vi "Constructor.vi"(8 "error in (no error)":errorcluster, 10 "Configuration.Application":enum16{"TC", "FP"}(ring), 11 "FP-TC-Shared in":refnum<class "FP-TC-Shared.lvclass">) -> (0 "error out":errorcluster, 3 "FP-TC-Shared out":refnum<class "FP-TC-Shared.lvclass">)   [LabVIEW 2019, in "FP-TC-Shared.lvclass"]
uses:
  FP-TC-Shared.lvclass
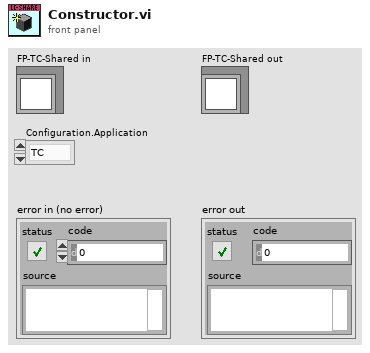
[diagram p1: front panel]
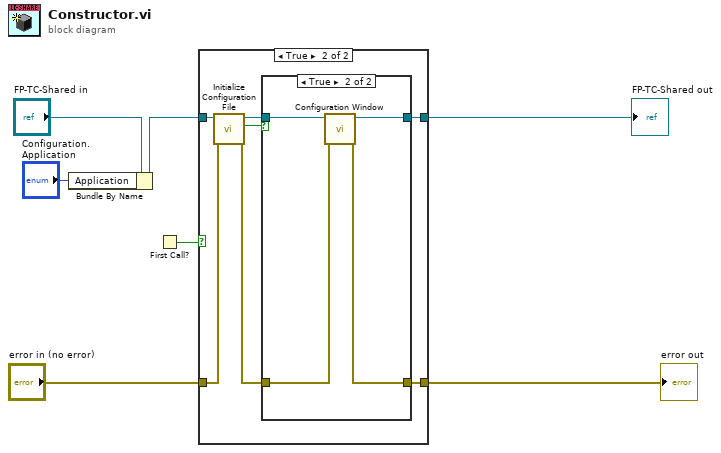
[diagram p0: block diagram]
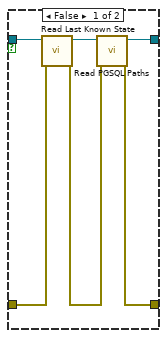
[diagram p3: hidden frame]
diagram:
  n1 = Bundle By Name(cluster="FP-TC-Shared in", "Application"="Configuration.Application") -> (w2:refnum<class "FP-TC-Shared.lvclass">)
  n2 = First Call?() -> (First Call?: T/F=w7:bool)
  n3 = case shown="True" w7 {
    tunnel: [w9 w16] -> w4
    tunnel: [w8 w15] -> w5
    tunnel: w2 -> [w8 w14]
    tunnel: "error in (no error)" -> [w9 w10]
    frame False {
    }
    frame True {
      n4 = call "Initialize Configuration File.vi"("error in (no error)"=w10, "FP-TC-Shared in"=w14) -> ("error out"=w11:errorcluster, "Last State Unknown"=w12:bool, "FP-TC-Shared out"=w13:refnum<class "FP-TC-Shared.lvclass">)  [unwired: 7 in]
      n5 = case shown="True" w12 {
        tunnel: [w21 w26] -> w15
        tunnel: w13 -> [w20 w23]
        tunnel: [w18 w24] -> w16
        tunnel: w11 -> [w17 w25]
        frame False {
          n6 = call "Read Last Known State.vi"("error in (no error)"=w17, "FP-TC-Shared in"=w20) -> ("error out"=w19:errorcluster, "FP-TC-Shared out"=w22:refnum<class "FP-TC-Shared.lvclass">)  [unwired: 8 in]
          n7 = call "Read PGSQL Paths.vi"("error in (no error)"=w19, "FP-TC-Shared in"=w22) -> ("error out"=w18:errorcluster, "FP-TC-Shared out"=w21:refnum<class "FP-TC-Shared.lvclass">)  [unwired: 8 in]
        }
        frame True {
          n8 = call-dynamic "Configuration Window.vi"("error in (no error)"=w25, "FP-TC-Shared"=w23) -> ("error out"=w24:errorcluster, "FP-TC-Shared out"=w26:refnum<class "FP-TC-Shared.lvclass">)  [unwired: 8 in]
        }
      }
    }
  }
  "FP-TC-Shared out" <- w5
  "error out" <- w4
